vi "Check if number is changing.vi"(8 "Shift in":T1, 11 "Number to check":i32) -> (0 "Shift out":T1, 3 "Number Changing":bool)   [LabVIEW 2013]
panel:
  in  "Miliseconds to wait for new number":u32=1000
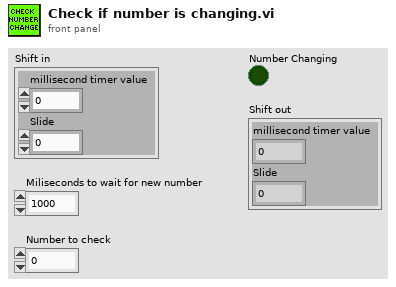
[diagram p1: front panel]
types:
  T1 = cluster{"millisecond timer value":u32, "Slide":i32}
  T2 = cluster{"millisecond timer value":u32, "Number to check":i32}
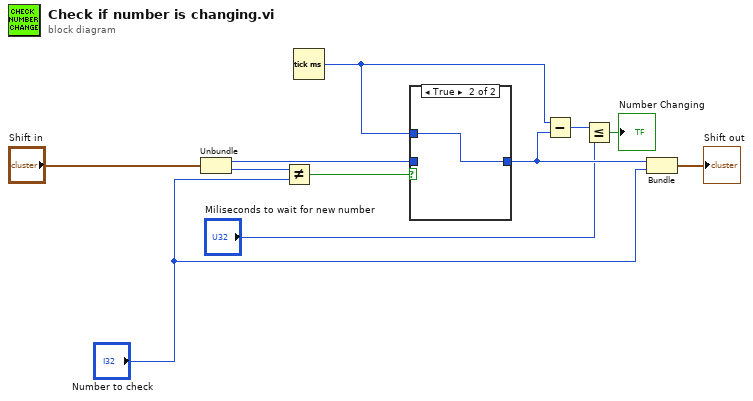
[diagram p0: block diagram]
diagram:
  n1 = Unbundle("Shift in") -> ("millisecond timer value"=w10:u32, "Slide"=w11:i32)
  n2 = Not Equal?(x=w11, y="Number to check") -> (x != y?=w1:bool)
  n3 = Tick Count (ms)() -> (millisecond timer value=w2:u32)
  n4 = case shown="True" w1 {
    tunnel: w2 -> [_ w13]
    tunnel: [w12 w13] -> w6
    tunnel: w10 -> [w12 _]
    frame False {
    }
    frame True {
    }
  }
  n5 = Subtract(x=w2, y=w6) -> (x-y=w3:u32)
  n6 = Less Or Equal?(x=w3, y="Miliseconds to wait for new number") -> (x <= y?=→"Number Changing":bool)
  n7 = Bundle("millisecond timer value"=w6, "Number to check"="Number to check") -> (→"Shift out":T2)  [unwired: 1 in]
